vi "Append Text Table to Report (wrap).vi"(0 "report in":refnum<class "NI_report.lvclass">, 1 "column width (1)":dbl=1.0 format="%.2f", 2 "measurement system":u16(ring)=2 caption="measurement system for column width (Default)" items=["US", "Metric", "Default"], 3 "MS Office parameters":T2, 5 "column headers":string[](array[string]), 7 "row headers":string[](array[string]), 9 "text data":string[][](array[string]), 11 "error in (no error)":errorcluster, 13 "separate page? (NO)":bool, 14 "show grid lines (YES)":bool=TRUE) -> (4 "report out":refnum<class "NI_report.lvclass">, 8 "range (wd) - start (xl)":T1, 10 "end (xl)":cluster{"row (xl) ":i32, "col (xl) ":i32}, 15 "error out":errorcluster)   [LabVIEW 2020, in "NI_report.lvclass"]
doc: "Appends a 2D array to a report as a table with the given column width. Wire data to the <B>text data</B> input to determine the polymorphic instance to use or manually select the instance."
uses:
  <vilib>/Utility/NIReport.llb/NI_report.lvclass
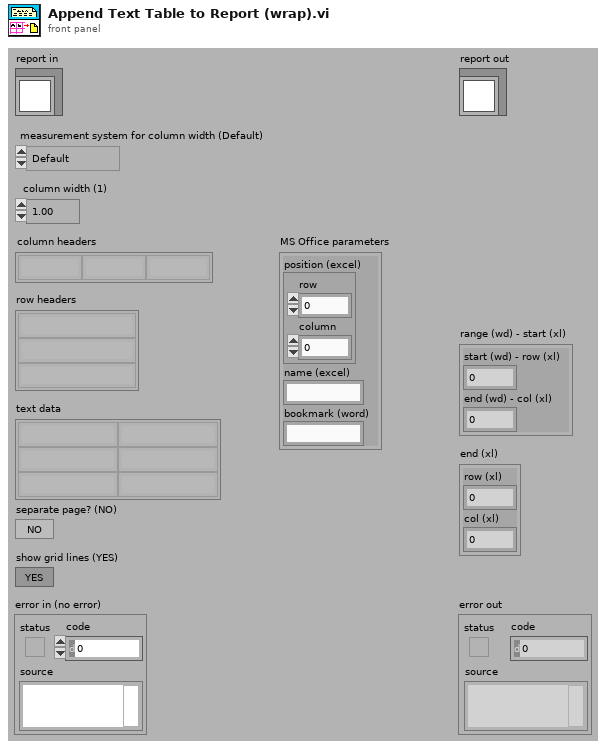
[diagram p1: front panel]
types:
  T1 = cluster{"start (wd) - row (xl) ":i32, "end (wd) - col (xl) ":i32}
  T2 = cluster{"position (excel)":cluster{"row":i32, "column":i32}, "name (excel)":string, "bookmark (word)":string}
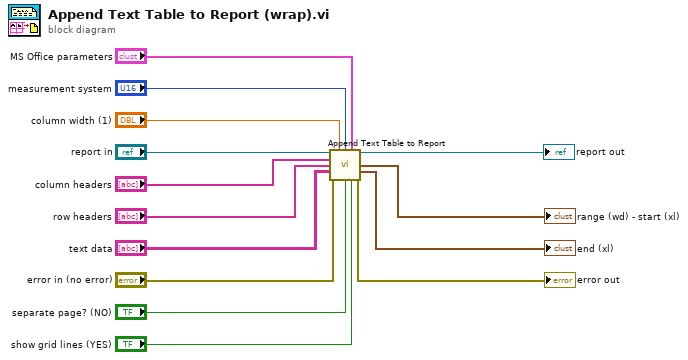
[diagram p0: block diagram]
diagram:
  n1 = call-dynamic "Append Text Table to Report.vi"("report in"="report in", "column width (1)"="column width (1)", "measurement system"="measurement system", "MS Office parameters"="MS Office parameters", "column headers"="column headers", "row headers"="row headers", "text data"="text data", "error in (no error)"="error in (no error)", "separate page? (NO)"="separate page? (NO)", "show grid lines (YES)"="show grid lines (YES)") -> ("report out"=→"report out":refnum<class "NI_report.lvclass">, "range (wd) - start (xl)"=→"range (wd) - start (xl)":T1, "end (xl)"=→"end (xl)":cluster{"row (xl) ":i32, "col (xl) ":i32}, "error out"=→"error out":errorcluster)  [unwired: 2 out]
